vi "Motor_SetSpeed.vi"(8 "error in":errorcluster, 9 "Speed":dbl min=-1.0 max=1.0, 10 "PWM_Channel":T1=1 items=["Invalid"=0, "PWM1"=1, "PWM2"=2, "PWM9"=9, "PWM10"=10]) -> (0 "error out":errorcluster)   [LabVIEW 2009, in "Motor.lvlib"]
uses:
  Motor.lvlib
  PWM/PWM_Name.ctl
  ControllerType.ctl
  PWM.lvlib
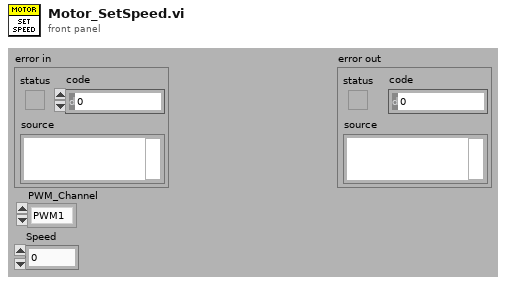
[diagram p1: front panel]
types:
  T1 = typedef "PWM.lvlib/PWM_Name.ctl" = u16
  T2 = typedef "Motor.lvlib/ControllerType.ctl" = u16
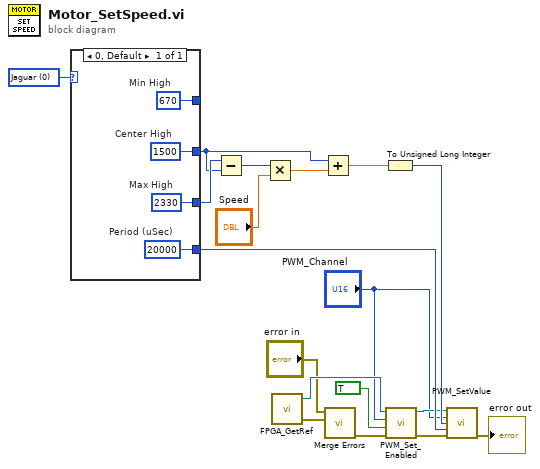
[diagram p0: block diagram]
diagram:
  w17 = T2 0 items=["Jaguar"] ("ControllerType")
  n1 = case shown="0, Default" w17 {
    tunnel: [w22] -> w10
    tunnel: [w21] -> _
    tunnel: [w20] -> w15
    tunnel: [w19] -> w16
    frame 0, Default {
      w19 = u32 2330  # Max High
      w20 = u32 1500  # Center High
      w21 = u32 670  # Min High
      w22 = u32 20000  # Period (uSec)
    }
  }
  n2 = Subtract(x=w16, y=w15) -> (x-y=w14:u32)
  n3 = Multiply(x=w14, y="Speed") -> (x*y=w12:dbl)
  n4 = call "FPGA_GetRef.vi"() -> ("error out"=w2:errorcluster, "FPGA_Ref"=w8:refnum<k20>)  [unwired: 1 in]
  n5 = Add(x=w15, y=w12) -> (x+y=w11:dbl)
  n6 = call <vilib>:"Merge Errors.vi"("error in 2 (no error)"=w2, "error in 1 (no error)"="error in") -> ("error out"=w1:errorcluster)  [unwired: 5 in]
  n7 = To Unsigned Long Integer(number=w11) -> (unsigned 32bit integer=w9:u32)
  n8 = call "PWM_Set_Enabled.vi"("error in"=w1, "Enable"=TRUE, "PWM_in"="PWM_Channel", "FPGA_Ref_in"=w8) -> ("error out"=w4:errorcluster, "FPGA_Ref_out"=w7:refnum<k20>)  [unwired: 5 in, 1 out]
  n9 = call "PWM_SetValue.vi"("FPGA_Ref_in"=w7, "PWM"="PWM_Channel", "High (uSec)"=w9, "Period (uSec)"=w10, "error in"=w4) -> ("error out"=→"error out":errorcluster)  [unwired: 9 in, 1 out]
